vi "Set Scaling (Linear).vi"(7 "Scaled Units":string, 8 "error in (no error)":errorcluster, 9 "Linear":T1={"Slope"=1.0, "Intercept"=0.0}, 10 "Scale Name":string, 11 "DAQmx(AI) in":refnum<class "DAQmx(AI).lvclass">) -> (0 "error out":errorcluster, 3 "DAQmx(AI) out":refnum<class "DAQmx(AI).lvclass">)   [LabVIEW 2019, in "DAQmx(AI).lvclass"]
uses:
  DAQmx(AI).lvclass
  Typedefs/Scaling(Linear)--Cluster.ctl
  Typedefs/ScalingType--Enum.ctl
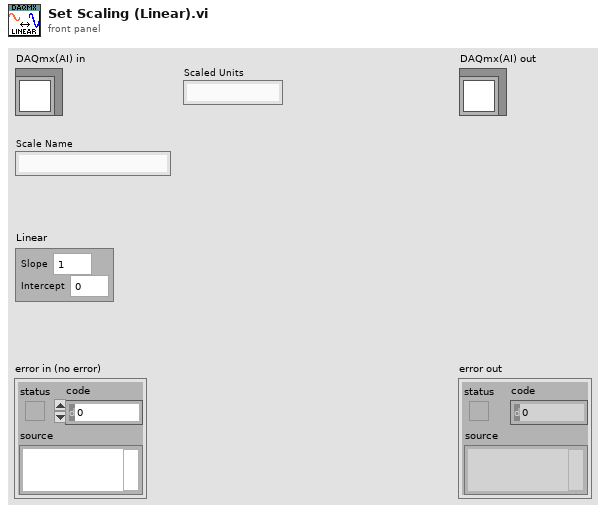
[diagram p1: front panel]
types:
  T1 = typedef "DAQmx(AI).lvclass/Scaling(Linear)--Cluster.ctl" = cluster{"Slope":dbl, "Intercept":dbl}
  T2 = typedef "DAQmx(AI).lvclass/ScalingType--Enum.ctl" = enum16{"No scaling", "Linear", "Map Range", "Polynomial", "Table"}
  T3 = typedef "DAQmx(AI).lvclass/Scaling--Cluster.ctl" = cluster{"Scale Name":string, "Scale Type":T2, "Scaled Units":string, "Linear":T1, "Map Range":T4, "Polynomial":T5, "Table":T6}
  T4 = typedef "DAQmx(AI).lvclass/Scaling(MapRange)--Cluster.ctl" = cluster{"Minimum":dbl, "Maximum":dbl}
  T5 = typedef "DAQmx(AI).lvclass/Scaling(Polynomial)--Cluster.ctl" = cluster{"forward coeff":dbl[], "reverse coeff":dbl[]}
  T6 = typedef "DAQmx(AI).lvclass/Scaling(Table)--Cluster.ctl" = cluster{"scaled values":dbl[], "pres-scaled values":dbl[]}
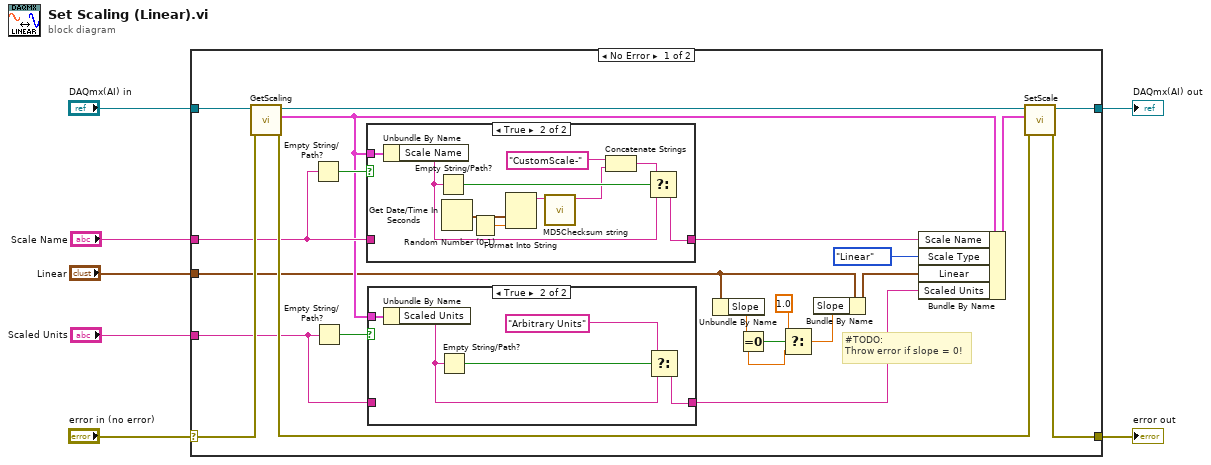
[diagram p0: block diagram]
diagram:
  n1 = case shown="No Error" "error in (no error)" {
    selector: "error in (no error)" -> [w24 w47]
    tunnel: [w27 w47] -> w6
    tunnel: [w28 w46] -> w4
    tunnel: "DAQmx(AI) in" -> [w26 w46]
    tunnel: "Scale Name" -> [w19 _]
    tunnel: "Scaled Units" -> [w14 _]
    tunnel: "Linear" -> [w13 _]
    frame No Error {
      # "#TODO: \nThrow error if slope = 0!"
      n2 = call "GetScaling.vi"("error in (no error)"=w24, "Subsystem"=w26) -> ("error out"=w21:errorcluster, "Scaling"=w16:T3, "Subsystem out"=w25:refnum<class "DAQmx(AI).lvclass">)  [unwired: 6 in, 1 out]
      n3 = Empty String/Path?(string/path=w19) -> (empty?=w20:bool)
      n4 = Empty String/Path?(string/path=w14) -> (empty?=w17:bool)
      n5 = case shown="True" w20 {
        tunnel: w16 -> [_ w45]
        tunnel: w19 -> [w35 _]
        tunnel: [w35 w42] -> w18
        frame False {
        }
        frame True {
          n6 = Unbundle By Name(w45) -> ("Scale Name"=w43:string)
          n7 = Empty String/Path?(string/path=w43) -> (empty?=w44:bool)
          n8 = Get Date/Time In Seconds() -> (seconds since 1Jan1904=w41:timestamp)
          n9 = Random Number (0-1)() -> (number: 0 to 1=w40:dbl)
          n10 = Format Into String(w41, w40) -> (resulting string=w39:string)  [unwired: 3 in, 1 out]
          n11 = call <vilib>:"MD5Checksum string.vi"("Message String"=w39) -> ("MD5 message-digest"=w37:string)  [unwired: 10 in]
          n12 = Concatenate Strings("CustomScale-" ("t"), w37) -> (w36:string)
          n13 = Select(t=w36, s=w44, f=w43) -> (s? t:f=w42:string)
        }
      }
      n14 = case shown="True" w17 {
        tunnel: w16 -> [_ w34]
        tunnel: w14 -> [w29 _]
        tunnel: [w29 w31] -> w15
        frame False {
        }
        frame True {
          n15 = Unbundle By Name(w34) -> ("Scaled Units"=w32:string)
          n16 = Empty String/Path?(string/path=w32) -> (empty?=w33:bool)
          n17 = Select(t="Arbitrary Units", s=w33, f=w32) -> (s? t:f=w31:string)
        }
      }
      n18 = Unbundle By Name(w13) -> ("Slope"=w8:dbl)
      n19 = Equal To 0?(x=w8) -> (x = 0?=w11:bool)
      n20 = Select(t=1.0, s=w11, f=w8) -> (s? t:f=w10:dbl)
      n21 = Bundle By Name(cluster=w13, "Slope"=w10) -> (w12:T1)
      n22 = Bundle By Name(cluster=w16, "Scale Name"=w18, "Scale Type"=ScalingType--Enum."Linear", "Linear"=w12, "Scaled Units"=w15) -> (w22:T3)
      n23 = call "SetScale.vi"("error in (no error)"=w21, "Scaling"=w22, "Subsystem"=w25) -> ("error out"=w27:errorcluster, "Subsystem out"=w28:refnum<class "DAQmx(AI).lvclass">)  [unwired: 7 in]
    }
    frame Error {
    }
  }
  "error out" <- w6
  "DAQmx(AI) out" <- w4
